vi "Main - Import Export EtherCAT Configuration.vi"(8 "error in":errorcluster, 11 "Node Ptr":T1 format="%.0x") -> (0 "error out":errorcluster)   [LabVIEW 2017, in "Scan Engine Custom Device.lvlib"]
uses:
  Scan Engine Custom Device.lvlib
  <vilib>/NI Veristand/Custom Device API/Custom Device Item Ref.ctl
  Globals/Scan Engine GUIDs.vi
  <vilib>/NI Veristand/Custom Device Tools/Custom Device Utility Library/Custom Device Utility Library.lvlib
  <vilib>/NI Veristand/Custom Device Tools/Custom Device Utility Library/NI VeriStand - Search for All Items by GUID.vi
  <vilib>/NI Veristand/Custom Device API/Custom Device API.lvlib
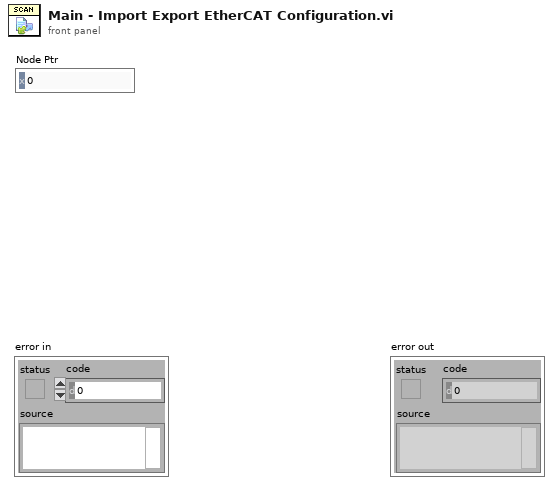
[diagram p1: front panel]
types:
  T1 = typedef "Custom Device API.lvlib/Custom Device Item Ref.ctl" = u64
  T2 = typedef "Scan Engine Custom Device.lvlib/Host - Import Export Action.ctl" = enum32{"Import", "Export", "Cancel"}
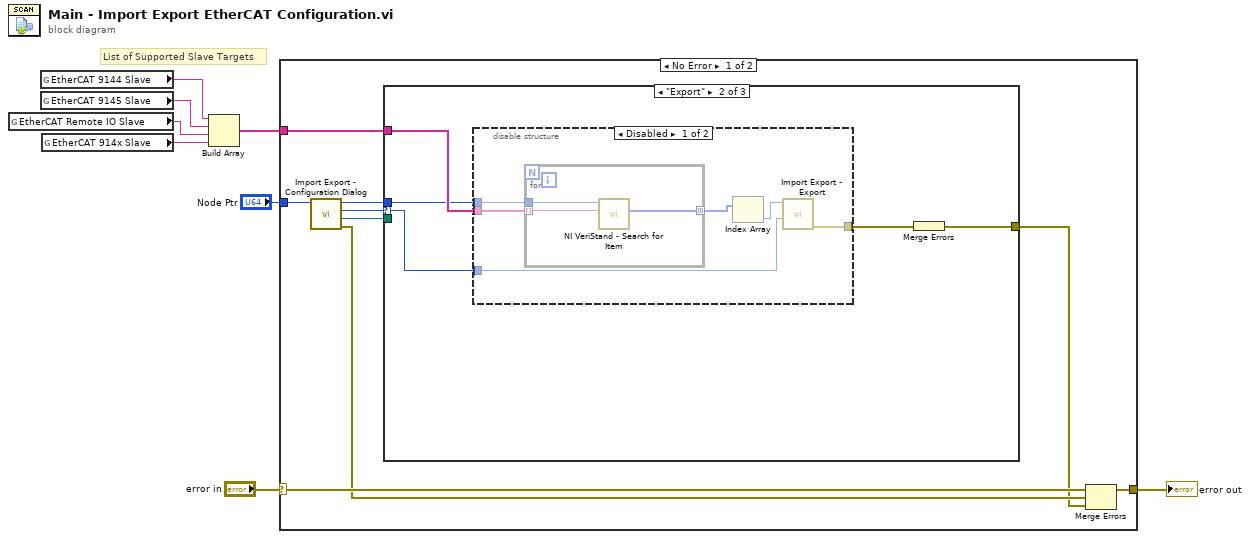
[diagram p0: block diagram]
diagram:
  # "List of Supported Slave Targets"
  n1 = global read "Scan Engine GUIDs.vi" "EtherCAT Remote IO Slave"() -> (w3:string)
  n2 = global read "Scan Engine GUIDs.vi" "EtherCAT 9144 Slave"() -> (w5:string)
  n3 = global read "Scan Engine GUIDs.vi" "EtherCAT 9145 Slave"() -> (w4:string)
  n4 = global read "Scan Engine GUIDs.vi" "EtherCAT 914x Slave"() -> (w2:string)
  n5 = Build Array(w5, w4, w3, w2) -> (w1:string[])
  n6 = case shown="No Error" "error in" {
    selector: "error in" -> [w17 w32]
    tunnel: [w12 w32] -> w7
    tunnel: "Node Ptr" -> [w16 _]
    tunnel: w1 -> [w9 _]
    frame No Error {
      n7 = call "Import Export - Configuration Dialog.vi"("Item Ref in"=w16) -> ("error out"=w11:errorcluster, "File Path"=w13:path, "Config Action"=w14:T2, "Item Ref out"=w15:T1)  [unwired: 6 in, 1 out]
      n8 = case shown="\"Export\"" w14 {
        selector: w14 -> [_ w20 _]
        tunnel: w15 -> [_ w18 _]
        tunnel: w13 -> [_ _ _]
        tunnel: [_ w19 _] -> w10
        tunnel: w9 -> [_ w21 _]
        frame "Import" {
        }
        frame "Export" {
          n9 = disable-structure shown="Disabled" {
            disable-tunnel: [w28 _] -> w22
            disable-tunnel: w18 -> [w27 _]
            disable-tunnel: w21 -> [w26 _]
            disable-tunnel: w20 -> [w23 _]
            frame Disabled {
              n10 = for {
                tunnel: w27 -> [w31]
                tunnel: w26 -> [w30] mode=indexing
                tunnel: [w29] -> w25 mode=concatenating
                n11 = call-poly <vilib>:"NI VeriStand - Search for Item.vi"("Item GUID"=w30, "Section Ref in"=w31) -> ("Item Refs"=w29:T1[])  [unwired: 6 in, 3 out]
              }
              n12 = Index Array(array=w25) -> (element=w24:T1)  [unwired: 1 in]
              n13 = call "Import Export - Export.vi"("Config Action"=w23, "Item Ref in"=w24) -> ("error out"=w28:errorcluster)  [unwired: 8 in, 1 out]
            }
            frame Enabled {
            }
          }
          n14 = Merge Errors(w22) -> (w19:errorcluster)
        }
        frame "Cancel", Default {
        }
      }
      n15 = Merge Errors(w17, w11, w10) -> (w12:errorcluster)
    }
    frame Error {
    }
  }
  "error out" <- w7
